vi "SendRRProtocol.vi"(7 "Send":bool, 9 "Initialize":bool, 10 "RR old":T1={"type"="roboRIO", "device"="", "name"="", "data"={">fpga_button"=FALSE, ">vin_voltage"=0.0, ">vin_current"=0.0, ">6v_voltage"=0.0, ">6v_current"=0.0, ">6v_active"=FALSE, ">6v_faults"=0.0, ">5v_voltage"=0.0, ">5v_current"=0.0, ">5v_active"=FALSE, ">5v_faults"=0.0, ">3v3_voltage"=0.0, ">3v3_current"=0.0, ">3v3_active"=FALSE, ">3v3_faults"=0.0}}, 11 "RR new":T1={"type"="roboRIO", "device"="", "name"="", "data"={">fpga_button"=FALSE, ">vin_voltage"=0.0, ">vin_current"=0.0, ">6v_voltage"=0.0, ">6v_current"=0.0, ">6v_active"=FALSE, ">6v_faults"=0.0, ">5v_voltage"=0.0, ">5v_current"=0.0, ">5v_active"=FALSE, ">5v_faults"=0.0, ">3v3_voltage"=0.0, ">3v3_current"=0.0, ">3v3_active"=FALSE, ">3v3_faults"=0.0}}) -> ()   [LabVIEW 2019]
uses:
  RoboRIO proto.ctl
  RoboRIO data proto.ctl
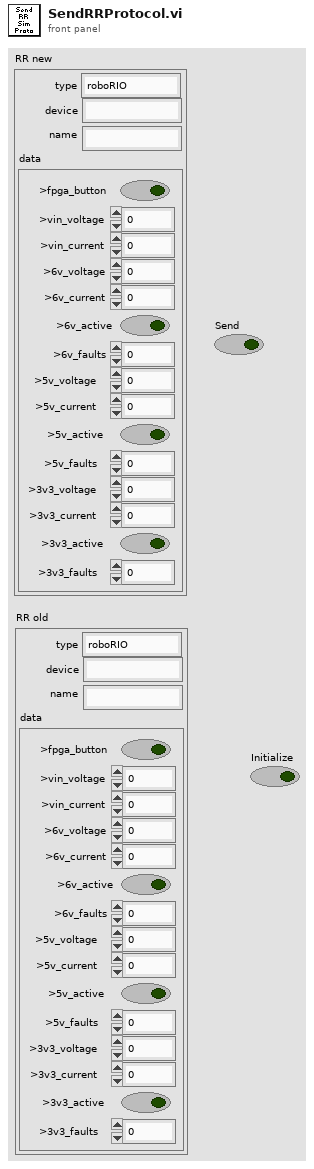
[diagram p1: front panel]
types:
  T1 = typedef "RoboRIO proto.ctl" = cluster{"type":string, "device":string, "name":string, "data":T2}
  T2 = typedef "RoboRIO data proto.ctl" = cluster{">fpga_button":bool, ">vin_voltage":dbl, ">vin_current":dbl, ">6v_voltage":dbl, ">6v_current":dbl, ">6v_active":bool, ">6v_faults":dbl, ">5v_voltage":dbl, ">5v_current":dbl, ">5v_active":bool, ">5v_faults":dbl, ">3v3_voltage":dbl, ">3v3_current":dbl, ">3v3_active":bool, ">3v3_faults":dbl}
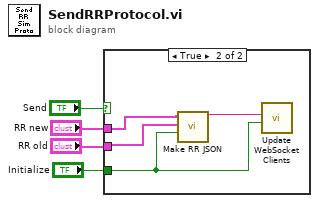
[diagram p0: block diagram]
diagram:
  n1 = case shown="True" "Send" {
    tunnel: "RR new" -> [_ w7]
    tunnel: "RR old" -> [_ w6]
    tunnel: "Initialize" -> [_ w5]
    frame False {
    }
    frame True {
      n2 = call "Make RR JSON.vi"("Force"=w5, "roboRIO prev"=w6, "roboRIO new"=w7) -> ("delta JSON"=w8:string)  [unwired: 8 in]
      n3 = call "Update WebSocket Clients.vi"("Initialize"=w5, "delta JSON"=w8) -> ()  [unwired: 10 in]
    }
  }
